vi "WriteData.vi"(8 "error in":errorcluster, 11 "File in":refnum<file>) -> (0 "error out":errorcluster, 3 "refnum out":refnum<file>)   [LabVIEW 2016]
uses:
  <vilib>/Rock Robotics/WPI/Utilities/WPI_GetSetVariantRefNum.vi
  Robot Global Data.vi
  Drive Base Class/DriveBase.lvclass
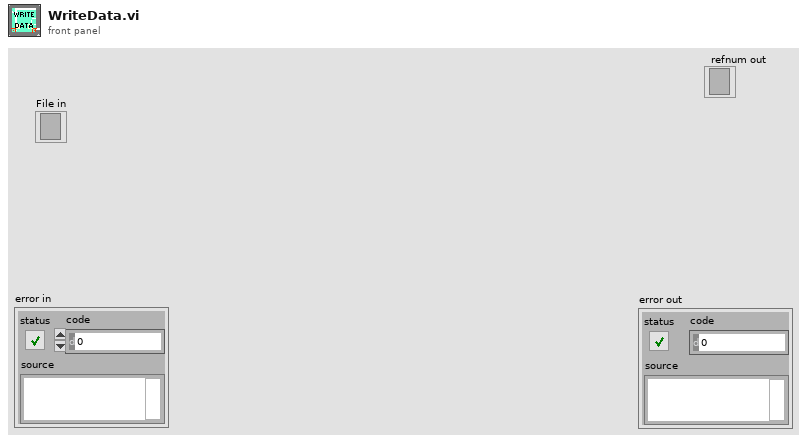
[diagram p1: front panel]
types:
  T1 = typedef "WPI_EncoderDevRef.ctl" = cluster{"DevStatus":errorcluster, "EncoderIndex":T2, "CounterIndex":T3, "DistancePerCount":dbl, "Decoding Type":T4}
  T2 = typedef "FPGA_EncoderIdx.ctl" = enum8{"Enc 0", "Enc 1", "Enc 2", "Enc 3", "Enc 4", "Enc 5", "Enc 6", "Enc 7", "Invalid"}
  T3 = typedef "FPGA_CounterCtrSystemIndex.ctl" = enum8{"Ctr 0", "Ctr 1", "Ctr 2", "Ctr 3", "Ctr 4", "Ctr 5", "Ctr 6", "Ctr 7", "Invalid"}
  T4 = typedef "WPI_EncoderType.ctl" = enum16{"1x", "2x", "4x"}
  T5 = typedef "WPI_PotentiometerDevRef.ctl" = cluster{"DevStatus":errorcluster, "Analog Channel":T6, "Invert Output":bool}
  T6 = typedef "FPGA_AIChannel.ctl" = enum8{"AI 0", "AI 1", "AI 2", "AI 3", "AI MXP 0", "AI MXP 1", "AI MXP 2", "AI MXP 3", "Invalid"}
  T7 = typedef "WPI_JoystickDevRef.ctl" = cluster{"Device":T8}
  T8 = typedef "WPI_JoystickDeviceEnum.ctl" = enum16{"USB 0", "USB 1", "USB 2", "USB 3", "USB 4", "USB 5"}
  T9 = typedef "WPI_DriverStationRobotMode2.ctl" = enum16{"Autonomous Disabled", "Autonomous Enabled", "Teleop Disabled", "Teleop Enabled", "Disconnected", "Finish", "Test Disabled", "Test Enabled", "Emergency Stopped"}
  T10 = cluster{"Yaw":dbl, "Roll":dbl, "Pitch":dbl, "Heading":dbl, "Fused Heading":dbl}
  T11 = cluster{"LinearAcceleration X":dbl, "LinearAcceleration Y":dbl, "LinearAcceleration Z":dbl}
  T12 = typedef "Z900_navX_Flags_OpStatusTypeDef.ctl" = u8
  T13 = typedef "Z900_navX_Flags_CalibrationStatusTypeDef.ctl" = u8
  T14 = cluster{"Update Rate Hz":u8, "Accelerometer Full-Scale Range":u8, "Gyro Full-Scale Range":u16, "OP Status":T12, "Calibration Status":T13, "Sensor Status":cluster{"MOVING":bool, "YAW_STABLE":bool, "MAG_DISTURBANCE":bool, "ALTITUDE_VALID":bool, "SEALEVEL_PRESS_SET":bool, "FUSED_HEADING_VALID":bool}, "Self Test Status":cluster{"Gyro Passed":bool, "Accel Passed":bool, "Mag Passed":bool, "Baro Passed":bool, "Complete":bool}}
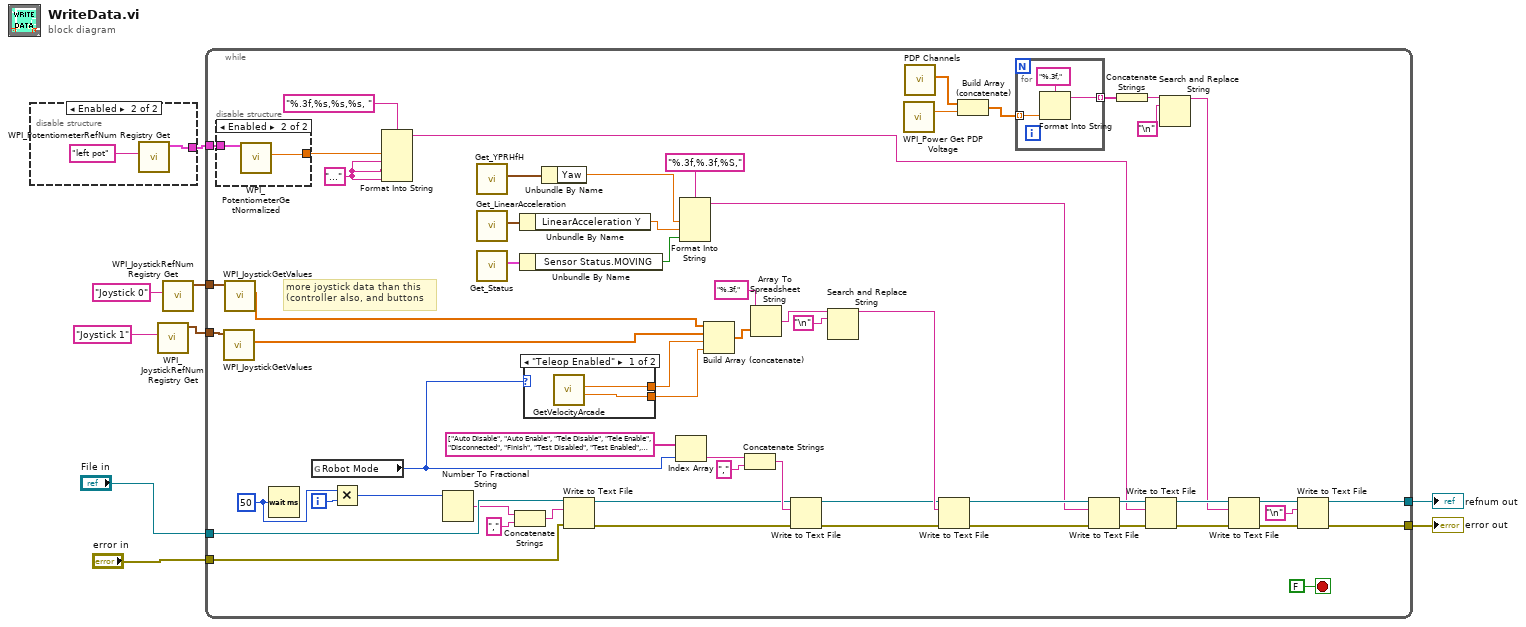
[diagram p0: block diagram]
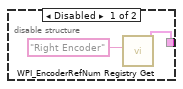
[diagram p2: hidden frame]
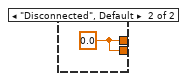
[diagram p3: hidden frame]
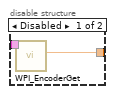
[diagram p4: hidden frame]
diagram:
  n1 = disable-structure shown="Enabled" {
    disable-tunnel: [w10 w12] -> w9
    frame Disabled {
      n2 = call <vilib>:"WPI_EncoderRefNum Registry Get.vi"("refnum name"="Right Encoder") -> ("EncoderDevRef"=w10:T1)  [unwired: 9 in, 1 out]
    }
    frame Enabled {
      n3 = call <vilib>:"WPI_PotentiometerRefNum Registry Get.vi"("refnum name"="left pot") -> ("PotDevRef"=w12:T5)  [unwired: 9 in, 1 out]
    }
  }
  n4 = call <vilib>:"WPI_JoystickRefNum Registry Get.vi"("refnum name"="Joystick 1") -> ("JoystickDevRef"=w1:T7)  [unwired: 9 in, 1 out]
  n5 = call <vilib>:"WPI_JoystickRefNum Registry Get.vi"("refnum name"="Joystick 0") -> ("JoystickDevRef"=w7:T7)  [unwired: 9 in, 1 out]
  n6 = while {
    tunnel: [w23] -> w4
    tunnel: [w22] -> w3
    tunnel: w9 -> [w52]
    tunnel: w7 -> [w51]
    tunnel: "File in" -> [w50]
    tunnel: "error in" -> [w49]
    tunnel: w1 -> [w48]
    i -> [w72]
    stop <- FALSE stop-if-true
    w20 = "..."
    w73 = u32 50 ("milliseconds to wait")
    # "more joystick data than this\n(controller also, and buttons"
    n7 = disable-structure shown="Enabled" {
      disable-tunnel: w52 -> [w81 w83]
      disable-tunnel: [w80 w82] -> w21
      frame Disabled {
        n8 = call <vilib>:"WPI_EncoderGet.vi"("EncoderDevRef"=w81) -> ("Distance"=w80:dbl)  [unwired: 5 in, 5 out]
      }
      frame Enabled {
        n9 = call <vilib>:"WPI_PotentiometerGetNormalized.vi"("PotDevRef"=w83) -> ("Normalized Value"=w82:dbl)  [unwired: 8 in, 2 out]
      }
    }
    n10 = call <vilib>:"WPI_JoystickGetValues.vi"("JoystickDevRef"=w48) -> ("Axes"=w26:dbl[])  [unwired: 6 in, 4 out]
    n11 = call <vilib>:"WPI_JoystickGetValues.vi"("JoystickDevRef"=w51) -> ("Axes"=w41:dbl[])  [unwired: 6 in, 4 out]
    n12 = Wait (ms)(milliseconds to wait=w73) -> ()  [unwired: 1 out]
    n13 = global read "Robot Global Data.vi" "Robot Mode"() -> (w29:T9)
    n14 = Multiply(x=w73, y=w72) -> (x*y=w71:u32)
    n15 = Format Into String(format string="%.3f,%s,%s,%s, ", w21, w20, w20, w20) -> (resulting string=w19:string)  [unwired: 2 in, 1 out]
    n16 = Number To Fractional String(number=w71) -> (F-format string=w46:string)  [unwired: 3 in]
    n17 = call <userlib>:"Get_YPRHfH.vi"() -> ("YRPHfH"=w62:T10)  [unwired: 11 in]
    n18 = call <userlib>:"Get_LinearAcceleration.vi"() -> ("Linear Acceleration"=w61:T11)  [unwired: 11 in]
    n19 = call <userlib>:"Get_Status.vi"() -> ("Status"=w56:T14)  [unwired: 11 in]
    n20 = Concatenate Strings(w46, "," ("string")) -> (w45:string)
    n21 = Unbundle By Name(w61) -> ("LinearAcceleration Y"=w33:dbl)
    n22 = Unbundle By Name(w56) -> ("Sensor Status.MOVING"=w32:bool)
    n23 = case shown="\"Teleop Enabled\"" w29 {
      tunnel: [w78 w79] -> w28
      tunnel: [w77 w79] -> w27
      frame "Teleop Enabled" {
        n24 = call "GetVelocityArcade.vi"() -> ("Y Axis"=w77:dbl, "X Axis"=w78:dbl)  [unwired: 9 in, 1 out]
      }
      frame "Disconnected", Default {
        w79 = 0.0 ("X Axis")
      }
    }
    n25 = Unbundle By Name(w62) -> ("Yaw"=w34:dbl)
    n26 = Write to Text File(file (use dialog)=w50, text=w45, error in=w49) -> (refnum out=w44:refnum<file>, error out=w43:errorcluster)  [unwired: 1 in, 1 out]
    n27 = Index Array(array=string[] ["Auto Disable", "Auto Enable", "Tele Disable", "Tele Enable", "Disconnected", "Finish", "Test Disabled", "Test Enabled", "Emergency Stopped"] ("Strings []"), index=w29) -> (element=w65:string)
    n28 = Format Into String(format string="%.3f,%.3f,%S,", w34, w33, w32) -> (resulting string=w30:string)  [unwired: 2 in, 1 out]
    n29 = Build Array (concatenate)(w41, w26, w28, w27) -> (w40:dbl[])
    n30 = Concatenate Strings(w65, "," ("string")) -> (w53:string)
    n31 = Array To Spreadsheet String(array=w40, 3:"%.3f," ("format string")) -> (spreadsheet string=w36:string)  [unwired: 1 in]
    n32 = Write to Text File(file (use dialog)=w44, text=w53, error in=w43) -> (refnum out=w25:refnum<file>, error out=w24:errorcluster)  [unwired: 1 in, 1 out]
    n33 = Search and Replace String(input string=w36, search string="\n") -> (result string=w35:string)  [unwired: 6 in, 3 out]
    n34 = call <vilib>:"WPI_Power Get PDP Voltage.vi"() -> ("voltage (V)"=w68:dbl)  [unwired: 14 in, 1 out]
    n35 = call "PDP Channels.vi"() -> ("appended array"=w17:dbl[])  [unwired: 11 in]
    n36 = Write to Text File(file (use dialog)=w25, text=w35, error in=w24) -> (refnum out=w60:refnum<file>, error out=w57:errorcluster)  [unwired: 1 in, 1 out]
    n37 = Build Array (concatenate)(w17, w68) -> (w16:dbl[])
    n38 = for {
      tunnel: w16 -> [w76] mode=indexing
      tunnel: [w74] -> w15 mode=indexing
      n39 = Format Into String(format string="%.3f,", w76) -> (resulting string=w74:string)  [unwired: 2 in, 1 out]
    }
    n40 = Write to Text File(file (use dialog)=w60, text=w30, error in=w57) -> (refnum out=w59:refnum<file>, error out=w58:errorcluster)  [unwired: 1 in, 1 out]
    n41 = Concatenate Strings(w15) -> (w14:string)
    n42 = Write to Text File(file (use dialog)=w59, text=w19, error in=w58) -> (refnum out=w64:refnum<file>, error out=w63:errorcluster)  [unwired: 1 in, 1 out]
    n43 = Search and Replace String(input string=w14, search string="\n") -> (result string=w38:string)  [unwired: 6 in, 3 out]
    n44 = Write to Text File(file (use dialog)=w64, text=w38, error in=w63) -> (refnum out=w55:refnum<file>, error out=w54:errorcluster)  [unwired: 1 in, 1 out]
    n45 = Write to Text File(file (use dialog)=w55, text="\n", error in=w54) -> (refnum out=w23:refnum<file>, error out=w22:errorcluster)  [unwired: 1 in, 1 out]
  }
  "refnum out" <- w4
  "error out" <- w3
